vi "execution class name.vi"(8 "error in":errorcluster, 11 "Central Error Handler configuration in":refnum<class "Central Error Handler configuration.lvclass">) -> (0 "error out":errorcluster, 2 "class name":string, 3 "Central Error Handler configuration out":refnum<class "Central Error Handler configuration.lvclass">)   [LabVIEW 2017, in "Central Error Handler configuration.lvclass"]
doc: "Provides an interface for determining the module runtime class associated with this module configuration. This class name can then be used to dynamically load or locate the runtime class for initialization purposes."
uses:
  Central Error Handler configuration.lvclass
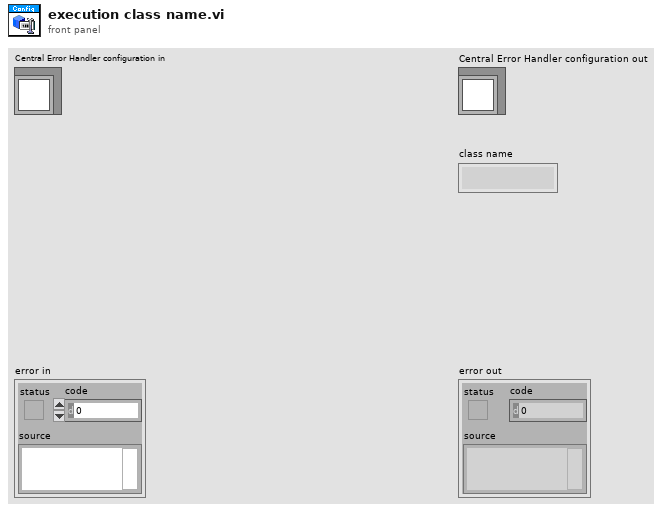
[diagram p1: front panel]
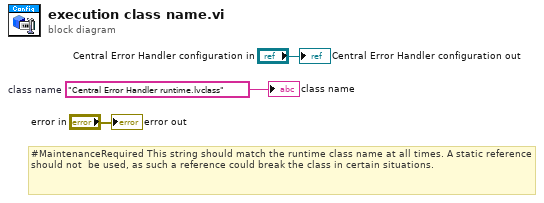
[diagram p0: block diagram]
diagram:
  w1 = "Central Error Handler runtime.lvclass"  # class name
  # "#MaintenanceRequired This string should match the runtime class name at all times. A static reference should not  be used, as such a reference could break the class in certain situations."
  "error out" <- "error in"
  "Central Error Handler configuration out" <- "Central Error Handler configuration in"
  "class name" <- w1
